vi "plc write string.vi"(8 "error in":errorcluster, 10 "value":string, 11 "addr,tag":T1 {"DataSocket Reference"."OnStatusUpdated" format="%.0x"; "DataSocket Reference"."OnDataUpdated" format="%.0x"}) -> (0 "error out":errorcluster)   [LabVIEW 2018]
uses:
  05.UserVI's/type defs/plc path and tag.ctl
  <vilib>/Platform/dataskt.llb/DataSocket Reference Type.ctl
  <vilib>/ethernetip/ethernetip.llb/EthernetIP Tag Write STRING.vi
  <vilib>/ethernetip/ethernetip.lvlib
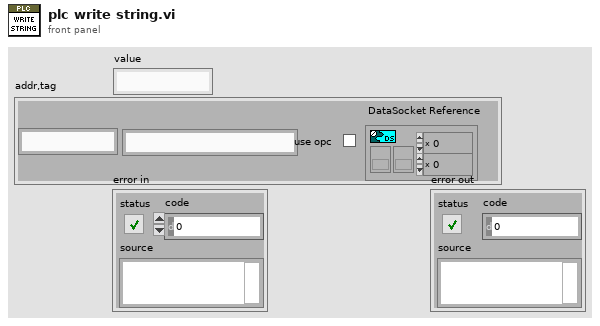
[diagram p1: front panel]
types:
  T1 = typedef "plc path and tag.ctl" = cluster{"Tag Name":string, "Network Path":string, "use opc":bool, "DataSocket Reference":T2}
  T2 = typedef "DataSocket Reference Type.ctl" = cluster{"CWDSLib._DCWDataSocket":refnum<k7>, "CWDSLib._DCWData":refnum<k7>, "OnDataUpdated":u32, "OnStatusUpdated":u32}
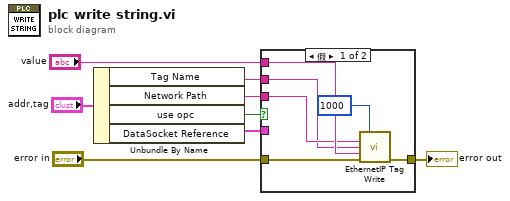
[diagram p0: block diagram]
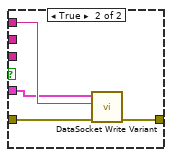
[diagram p2: hidden frame]
diagram:
  n1 = Unbundle By Name("addr,tag") -> ("Tag Name"=w3:string, "Network Path"=w4:string, "use opc"=w2:bool, "DataSocket Reference"=w1:T2)
  n2 = case shown="假" w2 {
    tunnel: "error in" -> [w14 w17]
    tunnel: [w13 w16] -> w6
    tunnel: "value" -> [w12 w18]
    tunnel: w4 -> [w11 _]
    tunnel: w3 -> [w10 _]
    tunnel: w1 -> [_ w15]
    frame False {
      n3 = call-poly <vilib>:"EthernetIP Tag Write.vi"("Timeout (ms)"=1000, "Network Path"=w11, "Tag Name"=w10, "Data"=w12, "error in"=w14) -> ("error out"=w13:errorcluster)  [unwired: 9 in, 1 out]
    }
    frame True {
      n4 = call <vilib>:"DataSocket Write Variant.vi"("error in (no error)"=w17, "Data"=w18, "DataSocket Reference In"=w15) -> ("error out"=w16:errorcluster)  [unwired: 5 in, 1 out]
    }
  }
  "error out" <- w6
